vi "VHRunVI.vi"(8 "error in (no error)":errorcluster) -> (0 "error out":errorcluster)   [LabVIEW 2013, in "VIHost.lvlib"]
uses:
  VIHost.lvlib
panel:
  out "Command line arguments":string[](array[string])
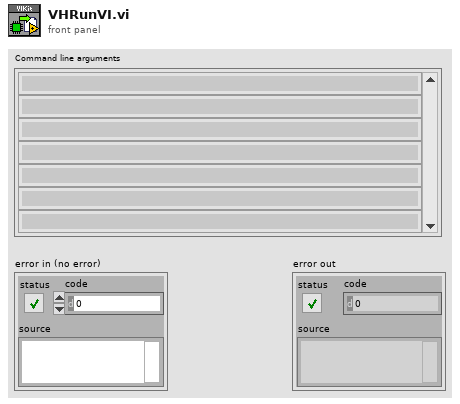
[diagram p1: front panel]
types:
  T1 = enum32{"Invalid", "Standard", "Closed", "Hidden", "Minimized", "Maximized"}
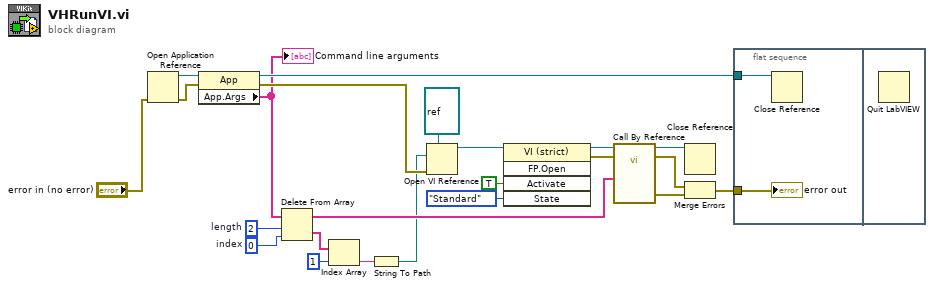
[diagram p0: block diagram]
diagram:
  w20 = 0  # index
  w22 = 2  # length
  n1 = Open Application Reference(8:"error in (no error)") -> (0:w13:errorcluster, 3:w14:refnum<vi>)  [unwired: 3 in]
  n2 = property class="App"(reference=w14, error in=w13) -> (reference out=w10:refnum<vi>, error out=w15:errorcluster, "App.Args"=w8:string[])
  "Command line arguments" <- w8
  n3 = Delete From Array "Delete From Array"(array=w8, length=w22, index=w20) -> (deleted portion=w21:string[], array with subset deleted=w18:string[])
  n4 = Index Array "Index Array"(array=w21, index=1) -> (element=w19:string)
  n5 = String To Path(string=w19) -> (path=w9:path)
  n6 = Open VI Reference(type specifier VI Refnum (for type only)=refnum<vi> refnum, vi path=w9, error in (no error)=w15) -> (vi reference=w5:refnum<vi>)  [unwired: 3 in, 1 out]
  n7 = invoke class="VI (strict)" method="FP.Open"(reference=w5, "Activate"=TRUE ("Activate?"), "State"=T1."Standard") -> (reference out=w3:refnum<vi>, error out=w4:errorcluster)  [unwired: 2 in, 3 out]
  n8 = call-by-ref "?"(reference=w3, error in=w4, "Paramters"=w18) -> (reference out=w2:refnum<vi>, error out=w1:errorcluster, 0:"error out"=w17:errorcluster)  [unwired: 10 in]
  n9 = Close Reference(reference=w2) -> ()  [unwired: 1 in, 1 out]
  n10 = Merge Errors(w1, w17) -> (w16:errorcluster)
  n11 = flat-sequence {
    tunnel: w16 -> [w25]
    tunnel: w10 -> [w24]
    frame #0 {
      n12 = Close Reference(reference=w24) -> ()  [unwired: 1 in, 1 out]
      "error out" <- w25
    }
    frame #1 {
      n13 = Quit LabVIEW() -> ()  [unwired: 1 in]
    }
  }
